vi "InitDispTable.vi"(8 "Error In":errorcluster, 11 "Table Display":refnum<vi>) -> (0 "Error Out":errorcluster)   [LabVIEW 2014]
uses:
  Controls/ColumnHeadersDisp.ctl
panel:
  in  "ColumnHeaders":T1
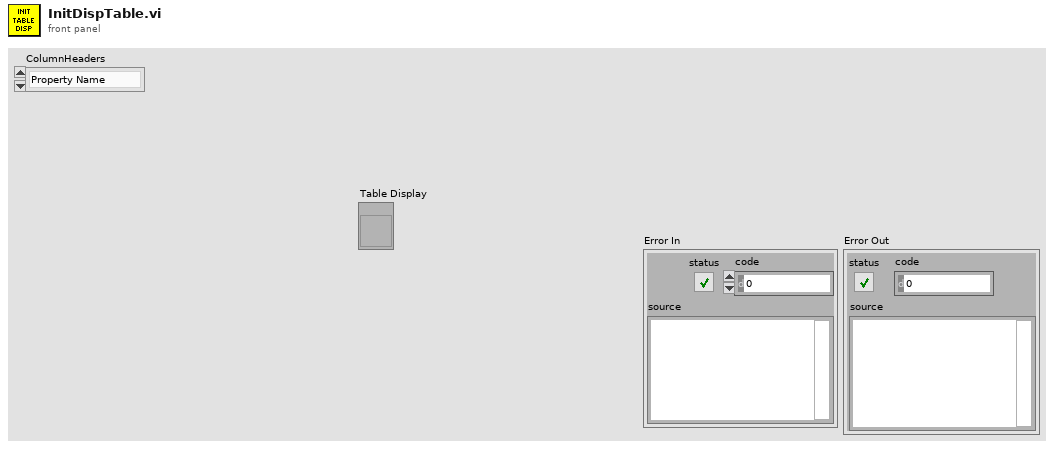
[diagram p1: front panel]
types:
  T1 = typedef "ColumnHeadersDisp.ctl" = enum16{"Property Name", "Value", "Unit"}
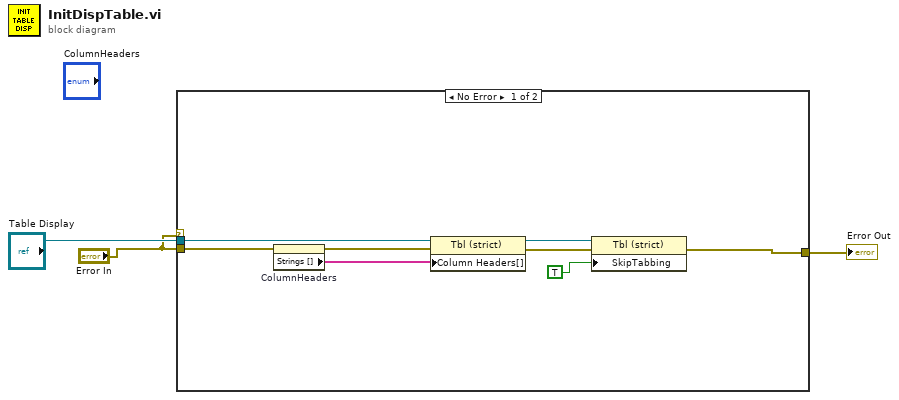
[diagram p0: block diagram]
diagram:
  n1 = case shown="No Error" "Error In" {
    tunnel: [w8 w12] -> w3
    tunnel: "Table Display" -> [w7 _]
    tunnel: "Error In" -> [w4 w12]
    frame No Error {
      n2 = property on="ColumnHeaders" class="Enum (strict)"(error in=w4) -> (error out=w5:errorcluster, "Strings []"=w6:string[])  [unwired: 1 in, 1 out]
      n3 = property on="Property Node" class="Tbl (strict)"(reference=w7, error in=w5, "Column Headers[]"=w6) -> (reference out=w11:refnum<vi>, error out=w10:errorcluster)
      n4 = property on="Property Node" class="Tbl (strict)"(reference=w11, error in=w10, "SkipTabbing"=TRUE ("Skip When Tabbing")) -> (error out=w8:errorcluster)  [unwired: 1 out]
    }
    frame Error {
    }
  }
  "Error Out" <- w3
